vi "8.2.vi"() -> ()   [LabVIEW 2020]
panel:
  out "Waveform Graph":T1(graph)
  in  "Folat 2":dbl
  in  "Numeric":i32
  in  "Cluster":T1
  in  "module path 3":path=path "C:/Users/Oliver/Videos/ylesanne2.py"
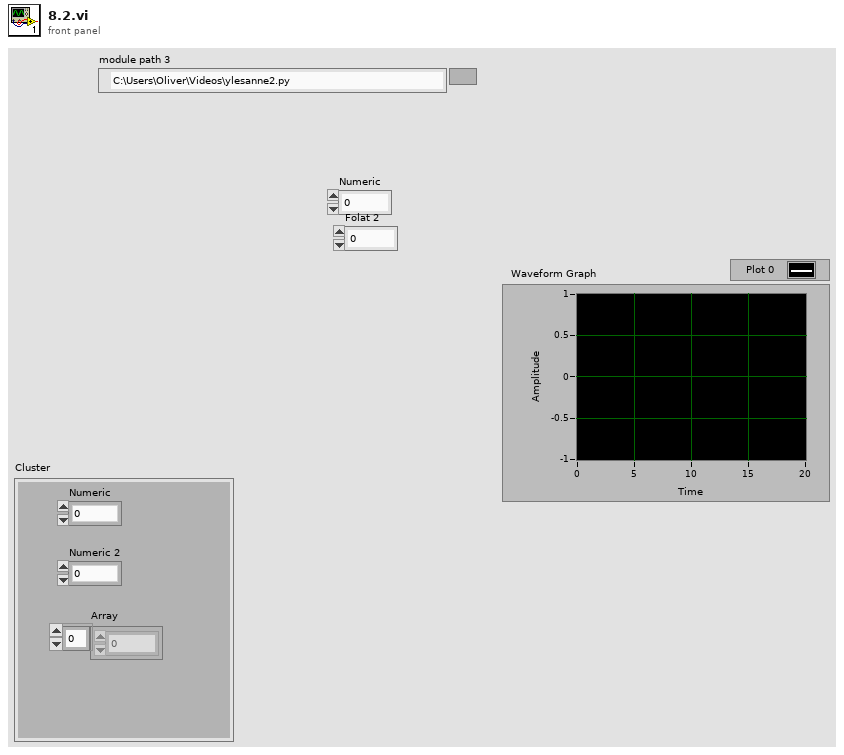
[diagram p1: front panel]
types:
  T1 = cluster{"Numeric":dbl, "Numeric 2":dbl, "Array":dbl[]}
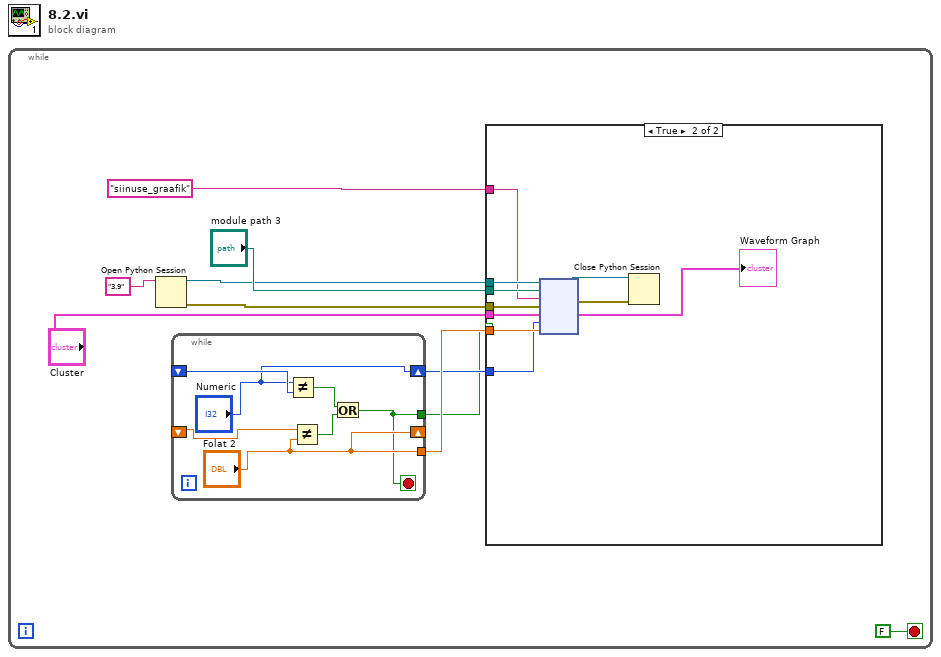
[diagram p0: block diagram]
diagram:
  n1 = while {
    stop <- FALSE stop-if-true
    n2 = Open Python Session(python version="3.9" ("Python version")) -> (session out=w8:refnum<k35>, error out=w7:errorcluster)  [unwired: 2 in]
    n3 = while {
      tunnel: ["Folat 2"] -> w4
      shift-right: ["Numeric"] -> w2
      shift-left: _ -> [w27]
      shift-right: ["Folat 2"] -> _
      shift-left: _ -> [w24]
      tunnel: [w21] -> w1
      stop <- w21 stop-if-true
      n4 = Not Equal?(x="Numeric", y=w27) -> (x != y?=w23:bool)
      n5 = Not Equal?(x=w24, y="Folat 2") -> (x != y?=w22:bool)
      n6 = Or(x=w23, y=w22) -> (x .or. y?=w21:bool)
    }
    n7 = case shown="True" w1 {
      tunnel: "module path 3" -> [_ w20]
      tunnel: w8 -> [_ w19]
      tunnel: w7 -> [_ w18]
      tunnel: "siinuse_graafik" ("function name") -> [_ w15]
      tunnel: "Cluster" -> [_ w14]
      tunnel: w4 -> [_ w12]
      tunnel: w2 -> [_ w11]
      frame False {
      }
      frame True {
        n8 = node(w19, w20, w15, w18, w14, w11, w12) -> (w17:refnum<k35>, w16:errorcluster, →"Waveform Graph":T1)  [unwired: 2 in, 2 out]
        n9 = Close Python Session(session in=w17, error in=w16) -> ()  [unwired: 1 out]
      }
    }
  }
